vi "Read2DdblArray.vi"(10 "Default":dbl[][](array[numeric]), 11 "Name":string) -> (3 "Read":dbl[][](array[numeric]))   [LabVIEW 2014]
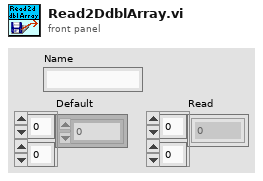
[diagram p1: front panel]
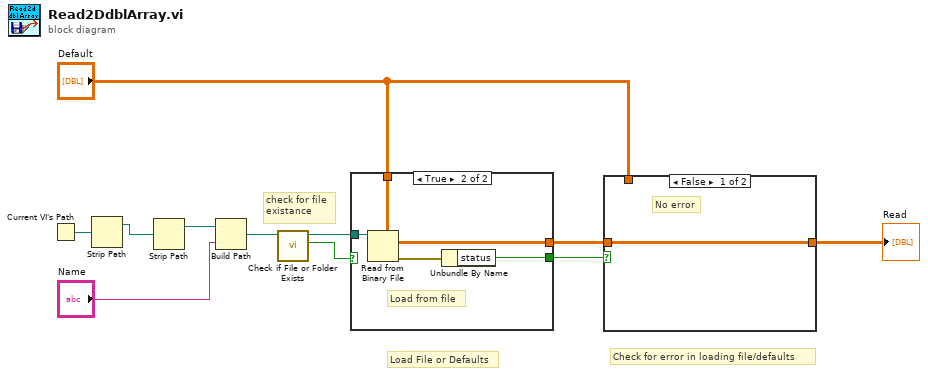
[diagram p0: block diagram]
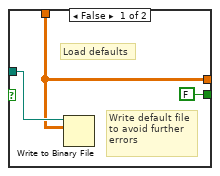
[diagram p3: hidden frame]
diagram:
  # "Check for error in loading file/defaults"
  # "Load File or Defaults"
  # "check for file\nexistance"
  n1 = Current VI's Path() -> (path=w10:path)
  n2 = Strip Path(path=w10) -> (stripped path=w11:path)  [unwired: 1 out]
  n3 = Strip Path(path=w11) -> (stripped path=w9:path)  [unwired: 1 out]
  n4 = Build Path(base path=w9, name or relative path="Name") -> (appended path=w8:path)
  n5 = call <vilib>:"Check if File or Folder Exists.vi"("path"=w8) -> ("file or folder exists?"=w7:bool, "dup path"=w6:path)  [unwired: 8 in, 1 out]
  n6 = case shown="True" w7 {
    tunnel: w6 -> [w13 w19]
    tunnel: [w12 w18] -> w4
    tunnel: [FALSE ("status") w16] -> w5
    tunnel: "Default" -> [w12 w15]
    frame False {
      # "Write default file\nto avoid further\nerrors"
      # "Load defaults"
      n7 = Write to Binary File(file (use dialog)=w13, data=w12) -> ()  [unwired: 4 in, 3 out]
    }
    frame True {
      # "Load from file"
      n8 = Read from Binary File(5:w15, 11:w19) -> (0:w17:errorcluster, 2:w18:dbl[][])  [unwired: 4 in, 2 out]
      n9 = Unbundle By Name(w17) -> ("status"=w16:bool)
    }
  }
  n10 = case shown="False" w5 {
    tunnel: [w20 w21] -> w1
    tunnel: w4 -> [w20 _]
    tunnel: "Default" -> [_ w21]
    frame False {
      # "No error"
    }
    frame True {
      # "Load defaults"
      # "Error when reading\nocurred"
    }
  }
  "Read" <- w1
